vi "RefTest.vi"() -> ()   [LabVIEW 2014]
panel:
  in  "String":string
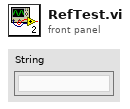
[diagram p1: front panel]
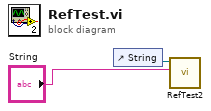
[diagram p0: block diagram]
diagram:
  n1 = control-ref of="String"() -> (w1:refnum<vi>)
  n2 = call "RefTest2.vi"("String"="String", "String in"=w1) -> ()  [unwired: 10 in]
